vi "Init Data.vi"(8 "error in (no error)":errorcluster, 10 "Data Object":refnum<class "Factory Plugin Framework.lvclass">, 11 "NF in":refnum<class "NF.lvclass">) -> (0 "error out":errorcluster, 3 "NF out":refnum<class "NF.lvclass">)   [LabVIEW 2018, in "NF.lvlib" / "NF.lvclass"]
uses:
  NF.lvclass
  Plugins/FPF.lvlibp/Factory Plugin Framework.lvclass
  Plugins/Measurement Interface.lvlibp/Measurement Interface.lvclass
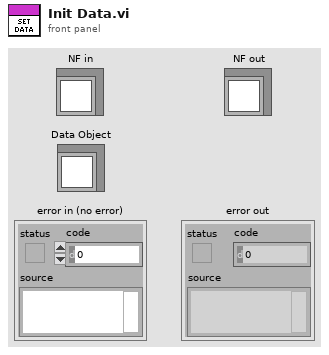
[diagram p1: front panel]
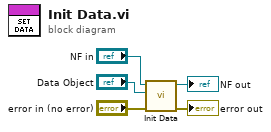
[diagram p0: block diagram]
diagram:
  n1 = call-parent "Init Data.vi"("error in (no error)"="error in (no error)", "Data Object"="Data Object", "Measurement Interface in"="NF in") -> ("error out"=→"error out":errorcluster, "Measurement Interface out"=→"NF out":refnum<class "NF.lvclass">)  [unwired: 7 in]
